vi "Main.vi"() -> ()   [LabVIEW 2017]
uses:
  <vilib>/Utility/error.llb/DialogType.ctl
  f8816c70-1855-4f5b-923a-05e49ab125c7.vi
  <vilib>/Utility/config.llb/Read Key (String).vi
  <vilib>/Utility/config.llb/Read Key (U32).vi
  <vilib>/Utility/config.llb/NI_LVConfig.lvlib
panel:
  out "Setting File Path":path=path "../data/Setting.txt"
  out "Error Out":errorcluster
  # "Note:- File Setting-\n1) e.g Application_path_To_Run D:\\Main_Application.exe\n2) Time should be in milisecond e.g Application_Delay_To_Run 1000\n3) Window servises for SQl Name e.g Services_Name_To_Check_Start_Status MySQL"
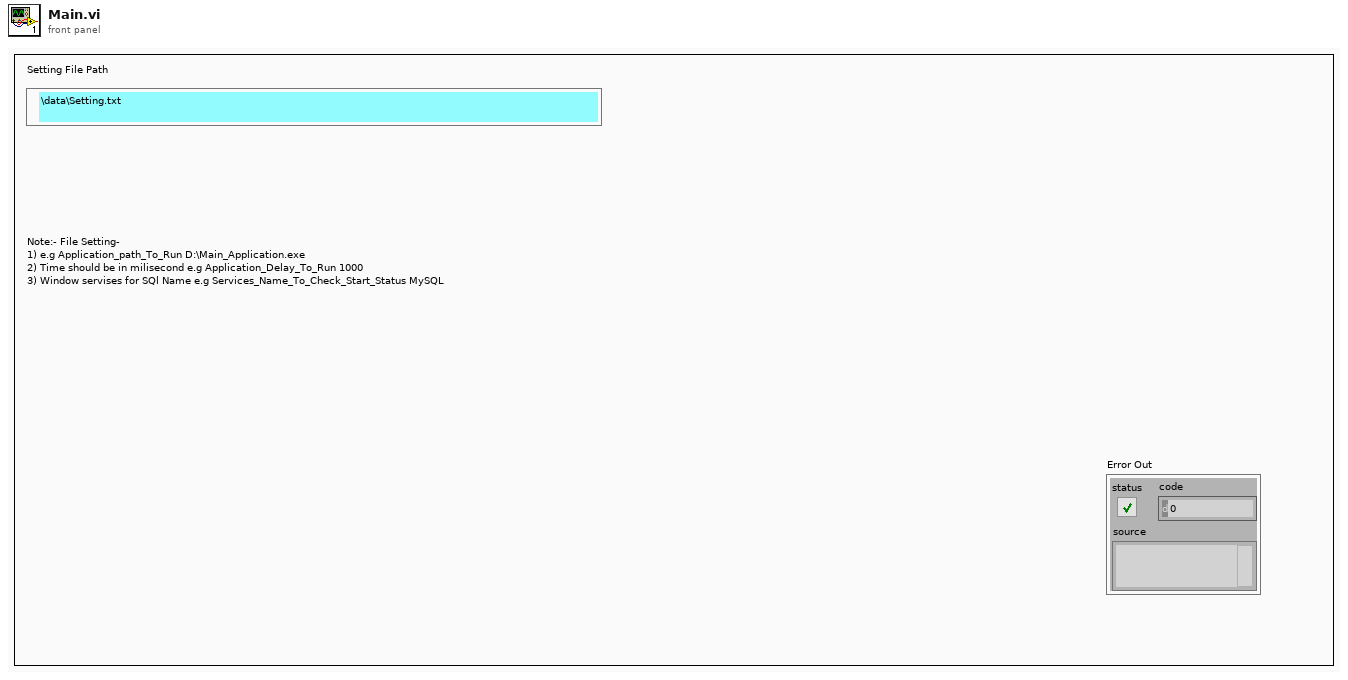
[diagram p1: front panel]
types:
  T1 = typedef "DialogType.ctl" = u16
  T2 = enum32{"invalid app kind", "Development System", "Run Time System", "Student Edition", "Embedded LabVIEW", "Evaluation", "Custom"}
  T3 = typedef "NI_LVConfig.lvlib/Config Data RefNum.ctl" = refnum<k1>
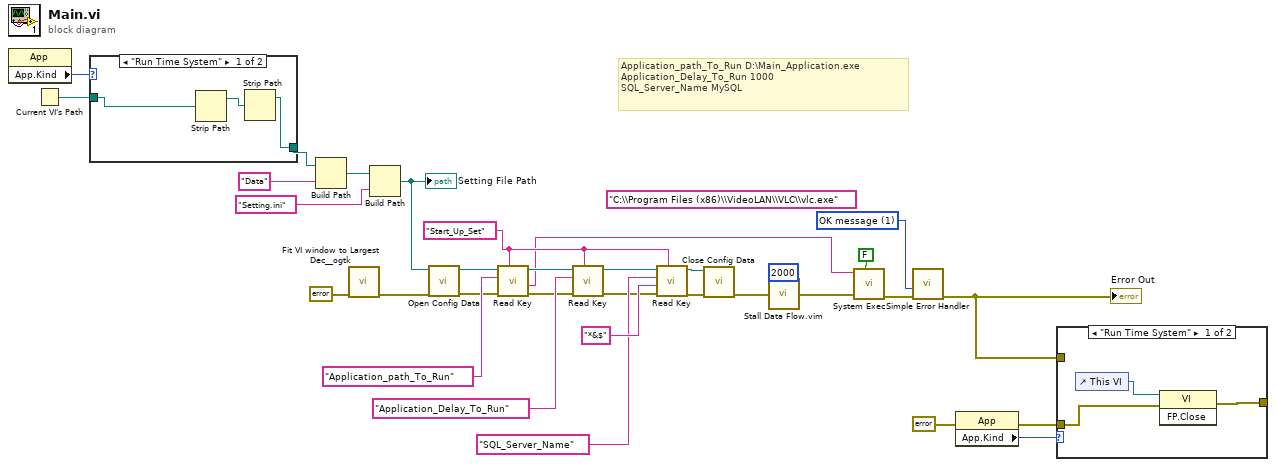
[diagram p0: block diagram]
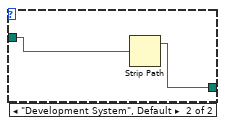
[diagram p3: hidden frame]
diagram:
  w10 = "Start_Up_Set" ("section")
  w21 = T1 1 items=["no dialog", "OK message", "continue or stop message", "OK message + warnings", "continue/stop + warnings"] ("type of dialog (OK msg:1)")
  (unwired) "C:\\Program Files (x86)\\VideoLAN\\VLC\\vlc.exe" ("command line")
  # "Application_path_To_Run D:\\Main_Application.exe\nApplication_Delay_To_Run 1000\nSQL_Server_Name MySQL"
  n1 = property class="App"() -> ("App.Kind"=w30:T2)  [unwired: 2 in, 2 out]
  n2 = Current VI's Path() -> (path=w31:path)
  n3 = case shown="\"Run Time System\"" w30 {
    tunnel: w31 -> [w35 w38]
    tunnel: [w34 w37] -> w28
    frame "Run Time System" {
      n4 = Strip Path(path=w35) -> (stripped path=w36:path)  [unwired: 1 out]
      n5 = Strip Path(path=w36) -> (stripped path=w34:path)  [unwired: 1 out]
    }
    frame "Development System", Default {
      n6 = Strip Path(path=w38) -> (stripped path=w37:path)  [unwired: 1 out]
    }
  }
  n7 = Build Path(base path=w28, name or relative path="Data") -> (appended path=w29:path)
  n8 = call <userlib>:"Fit VI window to Largest Dec__ogtk.vi"("error in (no error)"=errorcluster {"status"=FALSE, "code"=0, "source"=""}) -> ("error out"=w3:errorcluster)  [unwired: 5 in, 1 out]
  n9 = Build Path(base path=w29, name or relative path="Setting.ini") -> (appended path=w5:path)
  "Setting File Path" <- w5
  n10 = call <vilib>:"Open Config Data.vi"("error in (no error)"=w3, "configuration file path"=w5) -> ("error out"=w7:errorcluster, "refnum"=w6:T3)  [unwired: 7 in, 1 out]
  n11 = call-poly <vilib>:"Read Key.vi"("section"=w10, "error in (no error)"=w7, "key"="Application_path_To_Run", "refnum"=w6) -> ("error out"=w9:errorcluster, "value"=w4:string, "refnum out"=w8:T3)  [unwired: 4 in, 1 out]
  n12 = call-poly <vilib>:"Read Key.vi"("section"=w10, "error in (no error)"=w9, "key"="Application_Delay_To_Run", "refnum"=w8) -> ("error out"=w13:errorcluster, "refnum out"=w12:T3)  [unwired: 4 in, 2 out]
  n13 = call-poly <vilib>:"Read Key.vi"("section"=w10, "error in (no error)"=w13, "default value"="*&$", "key"="SQL_Server_Name", "refnum"=w12) -> ("error out"=w16:errorcluster, "refnum out"=w15:T3)  [unwired: 3 in, 2 out]
  n14 = call <vilib>:"Close Config Data.vi"("error in (no error)"=w16, "refnum"=w15) -> ("error out"=w2:errorcluster)  [unwired: 8 in, 1 out]
  n15 = call "Stall Data Flow.vim"("value in"=w2, "milliseconds to wait"=u32 2000) -> ("value out"=w1:errorcluster)  [unwired: 1 out]
  n16 = call <vilib>:"System Exec.vi"("wait until completion? (T)"=FALSE, "error in (no error)"=w1, "command line"=w4) -> ("error out"=w20:errorcluster)  [unwired: 5 in, 3 out]
  n17 = call <vilib>:"Simple Error Handler.vi"("type of dialog (OK msg:1)"=w21, "error in (no error)"=w20) -> ("error out"=w19:errorcluster)  [unwired: 3 in, 4 out]
  "Error Out" <- w19
  n18 = property class="App"(error in=errorcluster {"status"=FALSE, "code"=0, "source"=""} ("error in (no error)")) -> (error out=w23:errorcluster, "App.Kind"=w24:T2)  [unwired: 1 in, 1 out]
  n19 = case shown="\"Run Time System\"" w24 {
    tunnel: w23 -> [w40 w42]
    tunnel: [w39 w42] -> _
    tunnel: w19 -> [_ _]
    frame "Run Time System" {
      n20 = control-ref of="This VI"() -> (w41:refnum<vi>)
      n21 = invoke class="VI" method="FP.Close"(reference=w41, error in=w40) -> (error out=w39:errorcluster)  [unwired: 1 in, 2 out]
    }
    frame "Development System", Default {
    }
  }
